vi "log_loop.vi"(8 "error in (no error)":errorcluster, 10 "Log queue":refnum<queue>, 11 "Message Queues":T4) -> (0 "error out":errorcluster)   [LabVIEW 2013]
doc: "Message loop for handling messages pertaining to the acquisition of data from the hardware."
uses:
  queues/que_all_message_queues.ctl
  queues/que_message_cluster.ctl
  gui/type_def/general_and_device.ctl
  gui/type_def/general.ctl
  gui/type_def/device.ctl
  log_state.ctl
  queues/que_enqueue_message_single.vi
  <vilib>/Utility/error.llb/Error Cluster From Error Code.vi
  <vilib>/ErrorRing/Error Ring.xnode
panel:
  out "gral_&_device":T1={"general"={"file_ext"="0.0.0.0", "TCP port"=0, "#devices"=0, "log?"=FALSE, "tcp?"=FALSE, "language"="ENG"}, "eeg_device"={"name"="", "hardware"="", "image"="", "path"=path "", "extra"="", "channels"=""}}
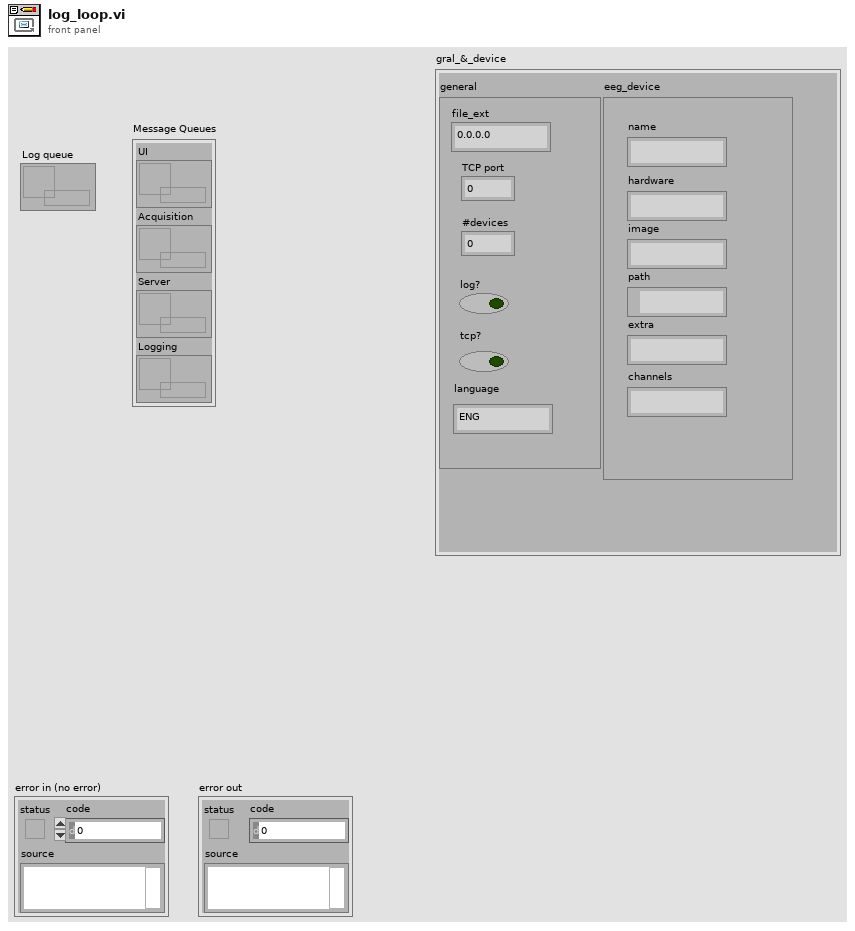
[diagram p1: front panel]
types:
  T1 = typedef "general_and_device.ctl" = cluster{"general":T2, "eeg_device":T3}
  T2 = typedef "general.ctl" = cluster{"file_ext":string, "TCP port":i32, "#devices":i32, "log?":bool, "tcp?":bool, "language":string}
  T3 = typedef "device.ctl" = cluster{"name":string, "hardware":string, "image":string, "path":path, "extra":string, "channels":string}
  T4 = typedef "que_all_message_queues.ctl" = cluster{"UI":refnum<queue>, "Acquisition":refnum<queue>, "Server":refnum<queue>, "Logging":refnum<queue>}
  T5 = typedef "log_state.ctl" = enum16{"Idle", "Logging"}
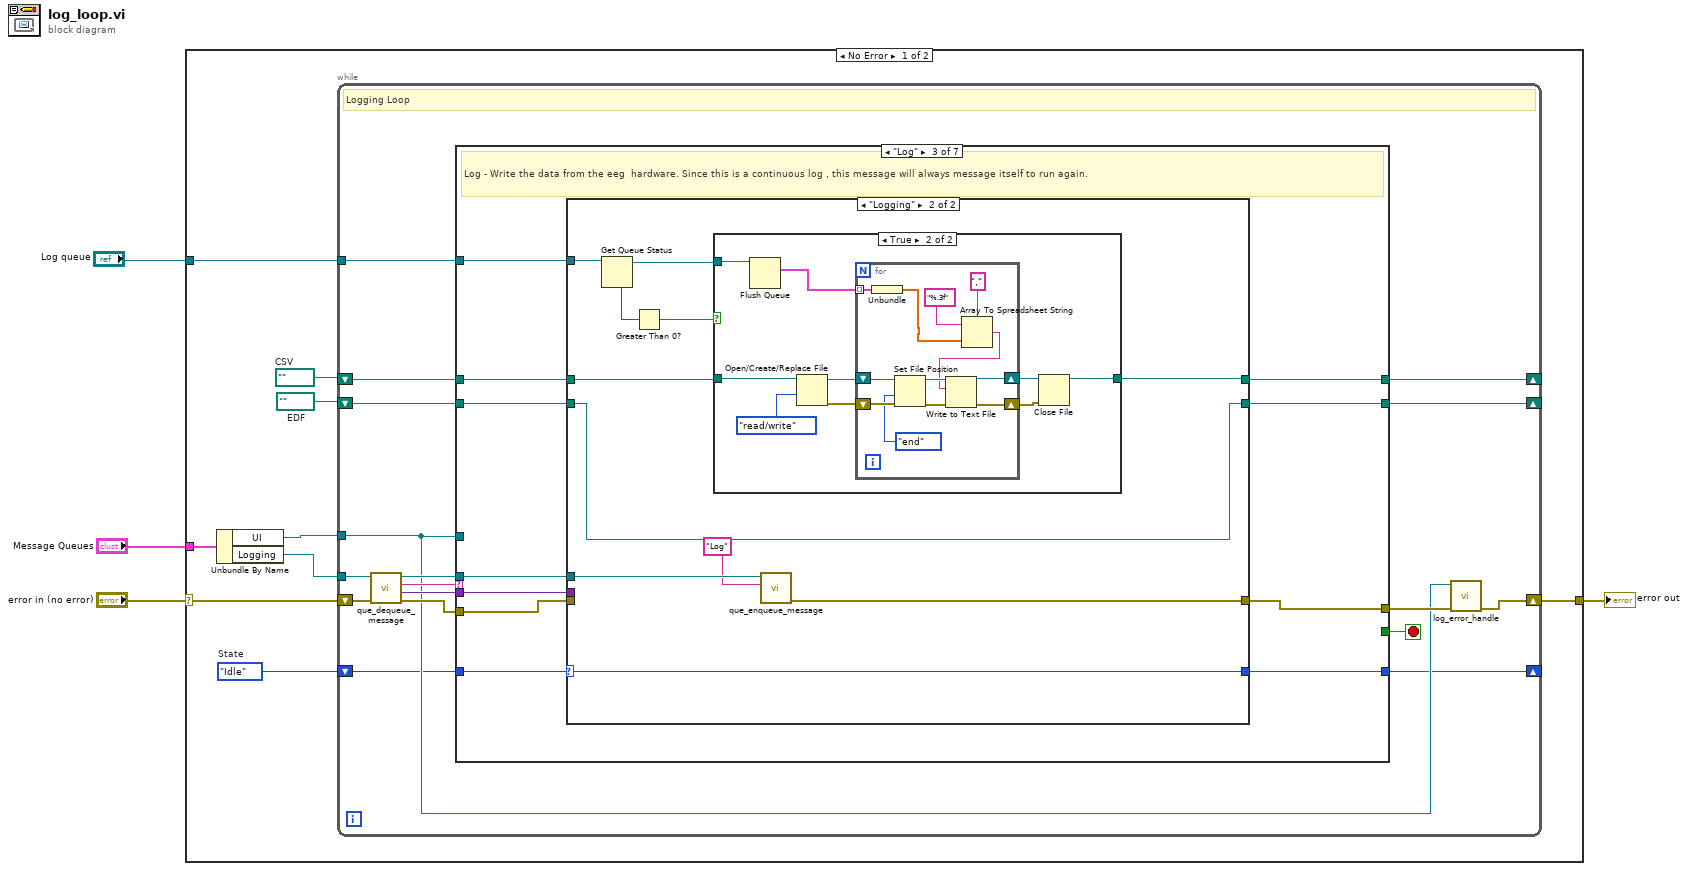
[diagram p0: block diagram]
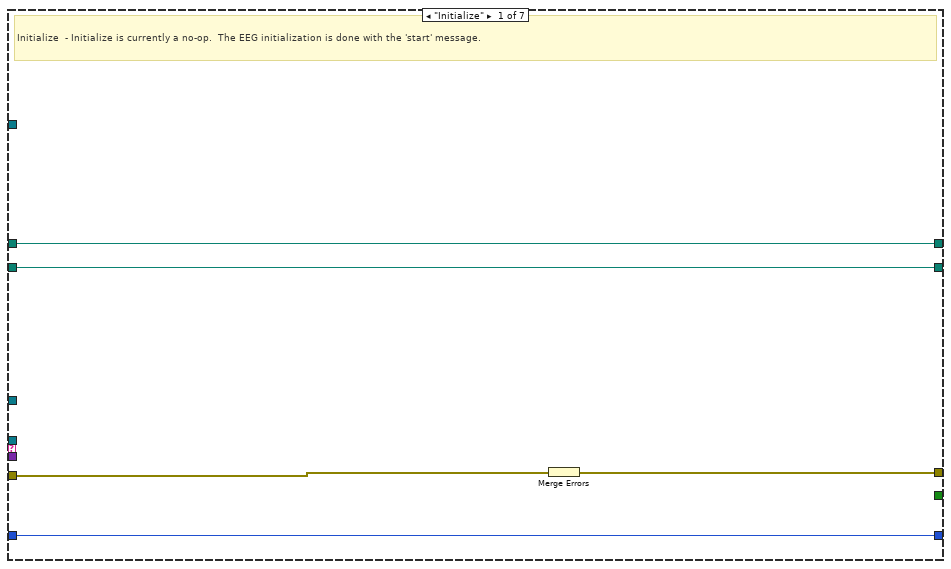
[diagram p2: hidden frame]
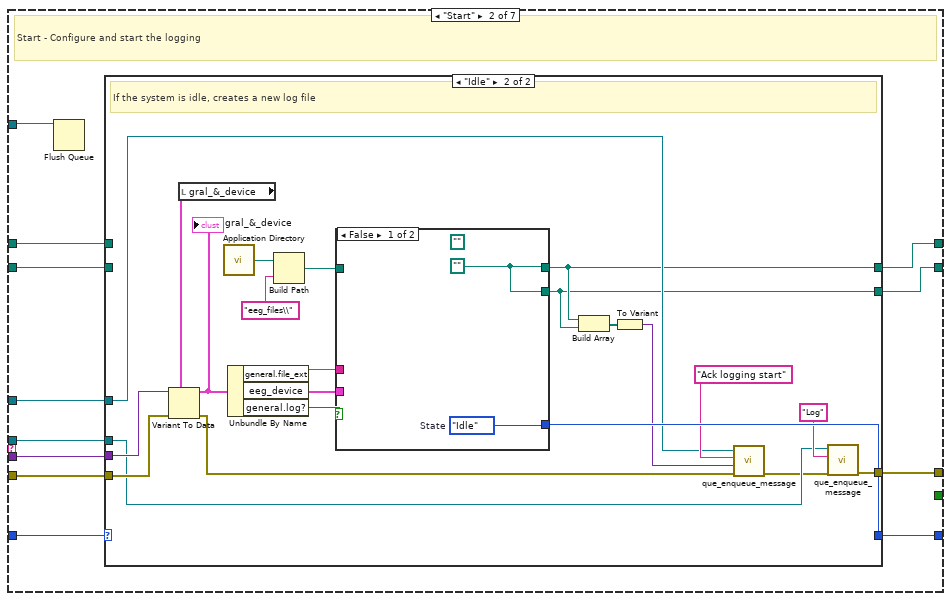
[diagram p3: hidden frame]
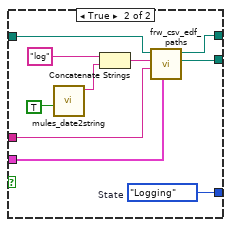
[diagram p5: hidden frame]
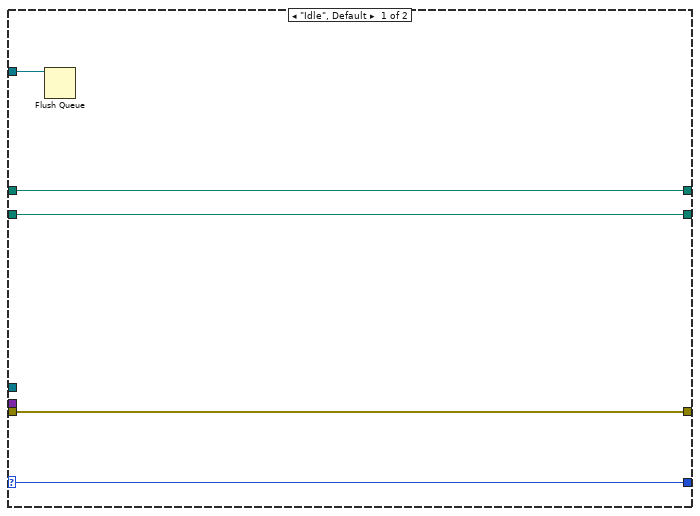
[diagram p6: hidden frame]
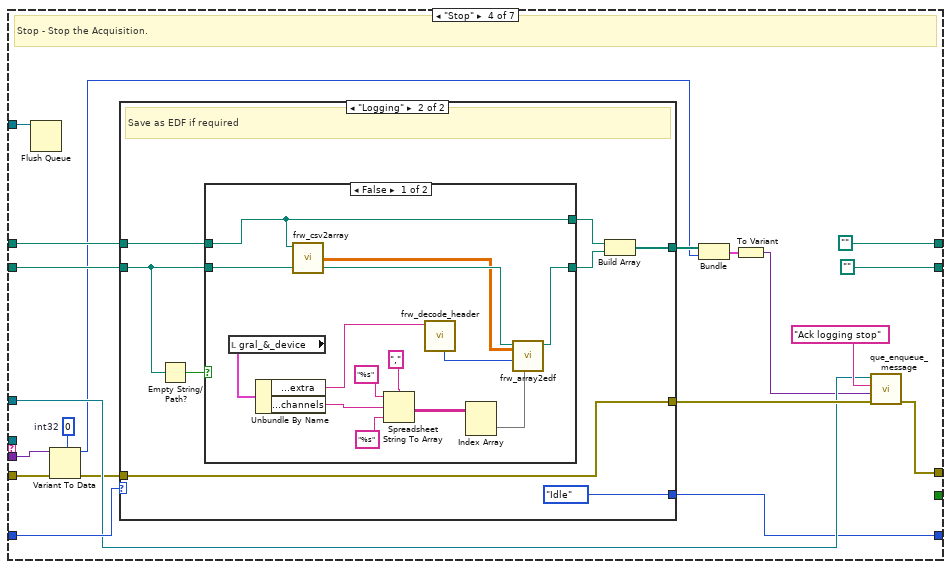
[diagram p8: hidden frame]
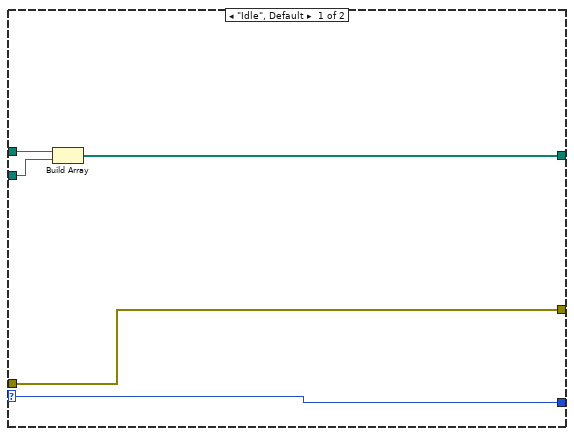
[diagram p9: hidden frame]
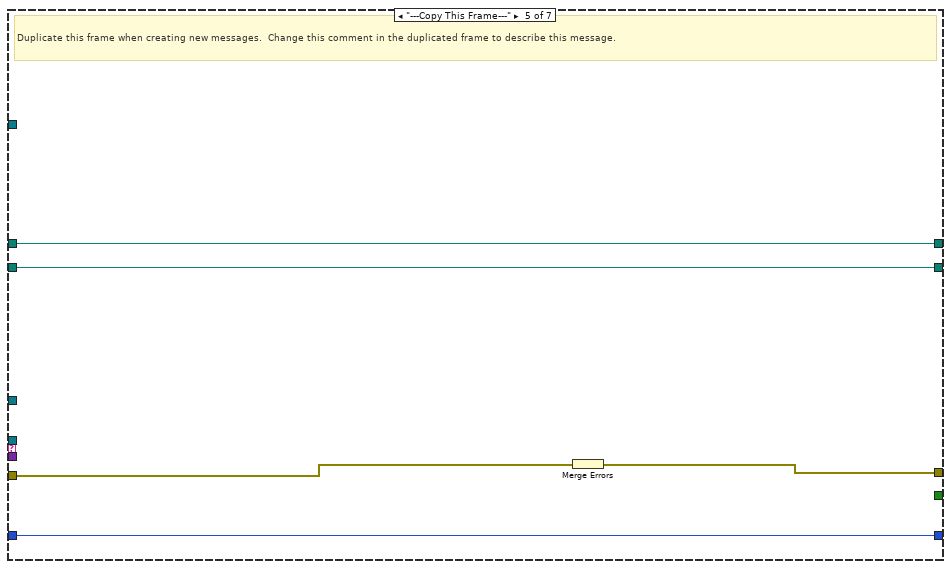
[diagram p11: hidden frame]
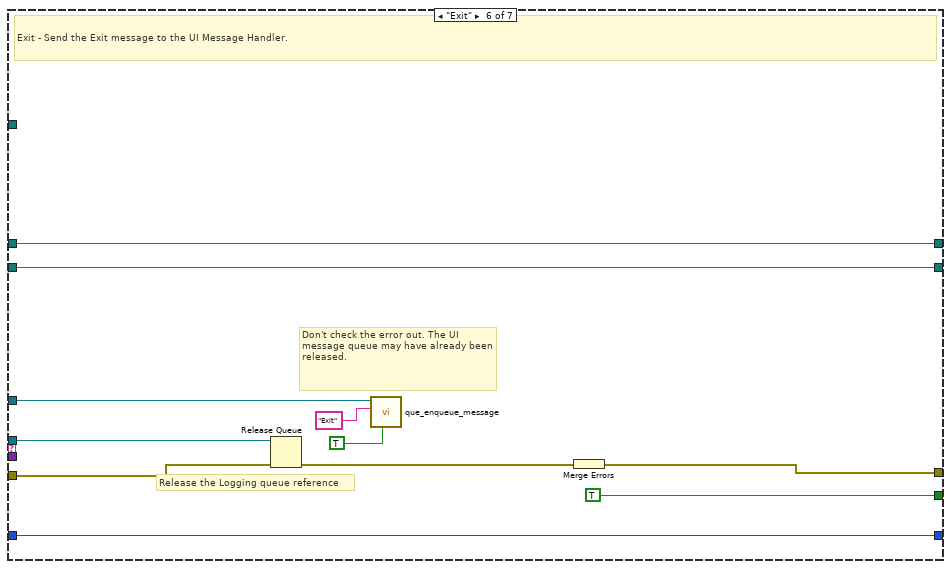
[diagram p12: hidden frame]
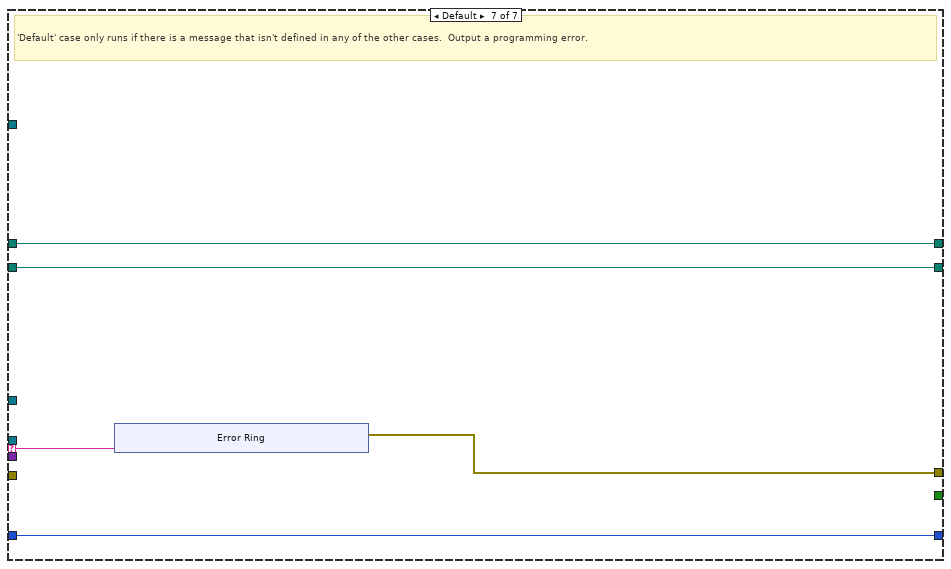
[diagram p13: hidden frame]
diagram:
  n1 = case shown="No Error" "error in (no error)" {
    selector: "error in (no error)" -> [w10 w210]
    tunnel: "Message Queues" -> [w13 _]
    tunnel: [w11 w210] -> w3
    tunnel: "Log queue" -> [w8 _]
    frame No Error {
      w5 = path ""  # EDF
      w7 = path ""  # CSV
      w6 = log_state."Idle"  # State
      n2 = Unbundle By Name(w13) -> ("UI"=w9:refnum<queue>, "Logging"=w12:refnum<queue>)
      n3 = while {
        tunnel: w12 -> [w25]
        shift-right: [w24] -> w11
        shift-left: w10 -> [w29]
        tunnel: w9 -> [w21]
        shift-right: [w20] -> _
        shift-left: w7 -> [w19]
        tunnel: w8 -> [w18]
        shift-right: [w16] -> _
        shift-left: w6 -> [w17]
        shift-right: [w14] -> _
        shift-left: w5 -> [w15]
        stop <- w30 stop-if-true
        # "Logging Loop"
        n4 = call "que_dequeue_message.vi"("error in (no error)"=w29, "Message Queue"=w25) -> ("error out"=w28:errorcluster, "Message Data"=w26:variant, "Message"=w27:string, "dup Message Queue"=w22:refnum<queue>)  [unwired: 6 in]
        n5 = case "Message Cases" shown="\"Log\"" w27 {
          selector: w27 -> [_ _ _ _ _ _ w200]
          tunnel: w22 -> [_ w47 w95 _ _ w190 _]
          tunnel: w28 -> [w34 w40 w94 w141 w186 w194 _]
          tunnel: [w35 w37 w96 w147 w185 w196 w201] -> w23
          tunnel: [_ _ _ _ _ TRUE _] -> w30
          tunnel: w26 -> [_ w44 w91 w140 _ _ _]
          tunnel: w21 -> [_ w41 _ w149 _ w195 _]
          tunnel: w17 -> [w33 w45 w92 w152 w184 w189 w202]
          tunnel: [w33 w46 w93 w148 w184 w189 w202] -> w16
          tunnel: [w32 w43 w87 path "" w183 w188 w199] -> w20
          tunnel: w19 -> [w32 w42 w90 w151 w183 w188 w199]
          tunnel: w18 -> [_ w36 w89 w135 _ _ _]
          tunnel: w15 -> [w31 w39 w88 w144 w182 w187 w198]
          tunnel: [w31 w38 w86 path "" w182 w187 w198] -> w14
          frame "Initialize" {
            # "Initialize  - Initialize is currently a no-op.  The EEG initialization is done with the 'start' message."
            n6 = Merge Errors(w34) -> (w35:errorcluster)
          }
          frame "Start" {
            # "Start - Configure and start the logging"
            n7 = Flush Queue(queue=w36) -> ()  [unwired: 1 in, 3 out]
            n8 = case shown="\"Idle\"" w45 {
              selector: w45 -> [w50 _]
              tunnel: [w51 w64] -> w37
              tunnel: w40 -> [w51 w72]
              tunnel: w47 -> [_ w60]
              tunnel: [w50 w66] -> w46
              tunnel: w44 -> [_ w73]
              tunnel: [w49 w55] -> w43
              tunnel: w42 -> [w49 _]
              tunnel: w41 -> [_ w57]
              tunnel: w39 -> [w48 _]
              tunnel: [w48 w54] -> w38
              frame "Logging" {
                # "The system is already acquiring. Ignore the \"Start\" message."
              }
              frame "Idle" {
                # "If the system is idle, creates a new log file"
                n9 = local read "gral_&_device"() -> (w71:T1)
                n10 = Variant To Data(error in=w72, type=w71, Variant=w73) -> (data=w70:T1, error out=w56:errorcluster)
                "gral_&_device" <- w70
                n11 = call <vilib>:"Application Directory.vi"() -> ("Application Directory"=w62:path)
                n12 = Unbundle By Name(w70) -> ("general.file_ext"=w67:string, "eeg_device"=w68:T3, "general.log?"=w69:bool)
                n13 = Build Path(base path=w62, name or relative path="eeg_files\\") -> (appended path=w61:path)
                n14 = case shown="False" w69 {
                  tunnel: w68 -> [_ w83]
                  tunnel: w67 -> [_ w85]
                  tunnel: [w74 w79] -> w55
                  tunnel: [w74 w78] -> w54
                  tunnel: [w75 w77] -> w66
                  tunnel: w61 -> [_ w76]
                  frame False {
                    w75 = log_state."Idle"  # State
                    w74 = path ""
                    (unwired) path ""
                  }
                  frame True {
                    w77 = log_state."Logging"  # State
                    n15 = call "mules_date2string.vi"("seconds?"=TRUE) -> ("date_time_string"=w81:string)  [unwired: 8 in, 2 out]
                    n16 = Concatenate Strings("log" ("string"), w81) -> (w80:string)
                    n17 = call "frw_csv_edf_paths.vi"("eeg_device"=w83, "file_extension"=w85, "filename"=w80, "directory path"=w76) -> ("path edf"=w78:path, "path csv"=w79:path)  [unwired: 6 in]
                  }
                }
                n18 = Build Array(w55, w54) -> (w53:path[])
                n19 = To Variant(anything=w53) -> (Variant=w52:variant)
                n20 = call-poly "que_enqueue_message.vi"("error in (no error)"=w56, "Message Data"=w52, "Message"="Ack logging start", "Message Queue"=w57) -> ("error out"=w58:errorcluster)  [unwired: 6 in, 1 out]
                n21 = call-poly "que_enqueue_message.vi"("error in (no error)"=w58, "Message"="Log", "Message Queue"=w60) -> ("error out"=w64:errorcluster)  [unwired: 7 in, 1 out]
              }
            }
          }
          frame "Log" {
            # "Log - Write the data from the eeg  hardware. Since this is a continuous log , this message will always message itself to run again."
            n22 = case shown="\"Logging\"" w92 {
              selector: w92 -> [w100 w112]
              tunnel: [w101 w111] -> w96
              tunnel: w95 -> [_ w110]
              tunnel: w94 -> [w101 _]
              tunnel: [w100 w112] -> w93
              tunnel: w91 -> [_ _]
              tunnel: w90 -> [w99 w103]
              tunnel: w89 -> [w97 w107]
              tunnel: w88 -> [w98 w108]
              tunnel: [w99 w102] -> w87
              tunnel: [w98 w108] -> w86
              frame "Idle", Default {
                # "Ignore \"Acquire\" messages when the acquisition is idle."
                n23 = Flush Queue(queue=w97) -> ()  [unwired: 1 in, 3 out]
              }
              frame "Logging" {
                # "Acquire more data while in the \"Acquiring\" state."
                n24 = Get Queue Status(queue=w107) -> (queue out=w105:refnum<queue>, # elements in queue=w106:i32)  [unwired: 2 in, 6 out]
                n25 = Greater Than 0?(x=w106) -> (x > 0?=w104:bool)
                n26 = case shown="True" w104 {
                  tunnel: w103 -> [w113 w119]
                  tunnel: [w113 w115] -> w102
                  tunnel: w105 -> [_ w122]
                  frame False {
                  }
                  frame True {
                    n27 = Flush Queue(queue=w122) -> (remaining elements=w121:cluster{dbl[]}[])  [unwired: 1 in, 2 out]
                    n28 = Open/Create/Replace File(file path (use dialog)=w119, access (0:read/write)=enum16{"read/write", "read-only", "write-only"}."read/write") -> (refnum out=w117:refnum<file>, error out=w118:errorcluster)  [unwired: 2 in, 3 out]
                    n29 = for {
                      tunnel: w121 -> [w134] mode=indexing
                      shift-right: [w129] -> w116
                      shift-left: w117 -> [w132]
                      shift-right: [w128] -> w114
                      shift-left: w118 -> [w133]
                      n30 = Unbundle(w134) -> (w125:dbl[])
                      n31 = Set File Position(refnum=w132, from (0:start)=enum16{"start", "end", "current"}."end", error in=w133) -> (refnum out=w130:refnum<file>, error out=w131:errorcluster)  [unwired: 1 in]
                      n32 = Array To Spreadsheet String(delimiter (Tab)=",", array=w125, 3:"%.3f" ("format string")) -> (spreadsheet string=w124:string)
                      n33 = Write to Text File(file (use dialog)=w130, text=w124, error in=w131) -> (refnum out=w129:refnum<file>, error out=w128:errorcluster)  [unwired: 2 out]
                    }
                    n34 = Close File(refnum=w116, error in=w114) -> (path=w115:path)  [unwired: 1 out]
                  }
                }
                n35 = call-poly "que_enqueue_message.vi"("Message"="Log", "Message Queue"=w110) -> ("error out"=w111:errorcluster)  [unwired: 8 in, 1 out]
              }
            }
          }
          frame "Stop" {
            w142 = 0  # int32
            # "Stop - Stop the Acquisition."
            n36 = Flush Queue(queue=w135) -> ()  [unwired: 1 in, 3 out]
            n37 = Variant To Data(error in=w141, type=w142, Variant=w140) -> (data=w139:i32, error out=w136:errorcluster)
            n38 = case shown="\"Logging\"" w152 {
              selector: w152 -> [w158 _]
              tunnel: [w157 w165] -> w150
              tunnel: w151 -> [w156 w160]
              tunnel: w136 -> [w157 w165]
              tunnel: [w158 log_state."Idle" ("State")] -> w148
              tunnel: w144 -> [w155 w164]
              tunnel: [w154 w159] -> w143
              frame "Idle", Default {
                n39 = Build Array(w156, w155) -> (w154:path[])
              }
              frame "Logging" {
                # "Save as EDF if required"
                n40 = Empty String/Path?(string/path=w164) -> (empty?=w163:bool)
                n41 = case shown="False" w163 {
                  tunnel: w164 -> [w170 w180]
                  tunnel: [w167 w180] -> w162
                  tunnel: [w169 w181] -> w161
                  tunnel: w160 -> [w169 w181]
                  frame False {
                    n42 = local read "gral_&_device"() -> (w179:T1)
                    n43 = Unbundle By Name(w179) -> ("eeg_device.extra"=w178:string, "eeg_device.channels"=w175:string)
                    n44 = call "frw_csv2array.vi"("file path"=w169) -> ("values"=w168:dbl[][])  [unwired: 7 in, 3 out]
                    n45 = Spreadsheet String To Array(delimiter (Tab)=",", format string="%s" ("delimiter (Tab)"), spreadsheet string=w175, array type (2D Dbl)="%s" ("delimiter (Tab)")) -> (array=w172:string[][])
                    n46 = call "frw_decode_header.vi"("header1"=w178) -> ("fs"=w177:i32)  [unwired: 5 in, 5 out]
                    n47 = Index Array(array=w172) -> (element=w171:string[])  [unwired: 2 in]
                    n48 = call "frw_array2edf.vi"("channel names"=w171, "fs"=w177, "2D array"=w168, "file path"=w170) -> ("path out"=w167:path)  [unwired: 6 in, 1 out]
                  }
                  frame True {
                  }
                }
                n49 = Build Array(w161, w162) -> (w159:path[])
              }
            }
            n50 = Bundle(w143, "int32"=w139) -> (w138:cluster{path[], "int32":i32})  [unwired: 1 in]
            n51 = To Variant(anything=w138) -> (Variant=w137:variant)
            n52 = call-poly "que_enqueue_message.vi"("error in (no error)"=w150, "Message Data"=w137, "Message"="Ack logging stop", "Message Queue"=w149) -> ("error out"=w147:errorcluster)  [unwired: 6 in, 1 out]
          }
          frame "---Copy This Frame---" {
            # "Duplicate this frame when creating new messages.  Change this comment in the duplicated frame to describe this message."
            n53 = Merge Errors(w186) -> (w185:errorcluster)
          }
          frame "Exit" {
            # "Don't check the error out. The UI message queue may have already been released."
            # "Release the Logging queue reference"
            # "Exit - Send the Exit message to the UI Message Handler."
            n54 = Release Queue(queue=w190, error in (no error)=w194) -> (error out=w191:errorcluster)  [unwired: 1 in, 2 out]
            n55 = call-poly "que_enqueue_message.vi"("Priority Message? (F)"=TRUE, "Message"="Exit", "Message Queue"=w195) -> ()  [unwired: 7 in, 2 out]
            n56 = Merge Errors(w191) -> (w196:errorcluster)
          }
          frame Default {
            # "'Default' case only runs if there is a message that isn't defined in any of the other cases.  Output a programming error."
            n57 = xnode "Error Ring"("parameter 0"=w200) -> ("error out"=w201:errorcluster)
          }
        }
        n58 = call "log_error_handle.vi"("error in (no error)"=w23, "Message Queue"=w21) -> ("dup error in"=w24:errorcluster)  [unwired: 8 in, 1 out]
      }
    }
    frame Error {
    }
  }
  "error out" <- w3
